vi "2. OCR.vi"() -> ()   [LabVIEW 2019]
doc: "c 2020 ReMiSYS All rights reserved."
panel:
  out "Image 2":T1(plugin-control)
  out "Data":string
  out "Image":T1(plugin-control)
  in  "Stop Button":bool
  # "c 2021 ReMiSYS All rights reserved."
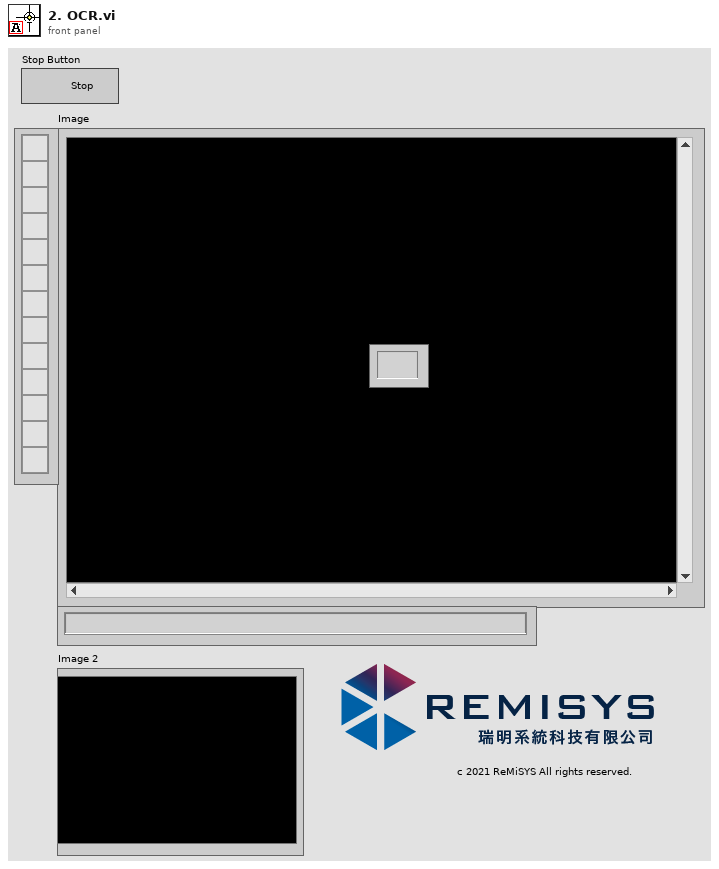
[diagram p1: front panel]
types:
  T1 = typedef "IMAQ Image.ctl" = refnum<image>
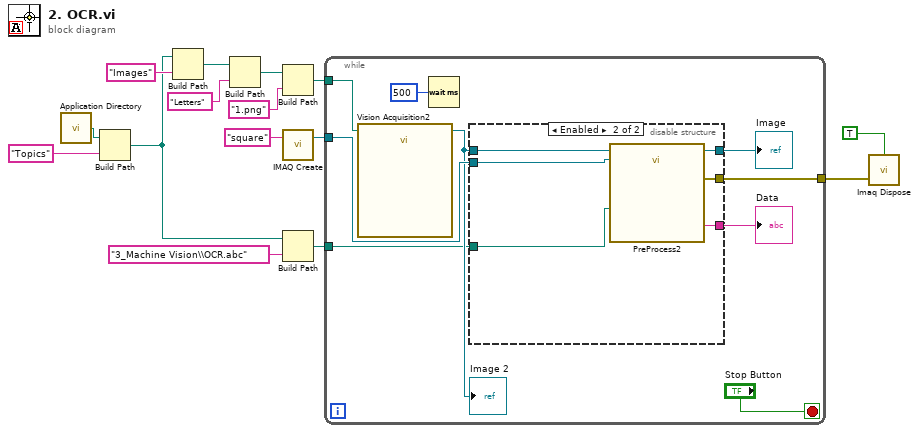
[diagram p0: block diagram]
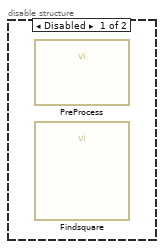
[diagram p2: hidden frame]
diagram:
  n1 = call <vilib>:"Application Directory.vi"() -> ("Application Directory"=w4:path)
  n2 = Build Path(base path=w4, name or relative path="Topics") -> (appended path=w1:path)
  n3 = Build Path(base path=w1, name or relative path="Images") -> (appended path=w8:path)
  n4 = Build Path(base path=w8, name or relative path="Letters") -> (appended path=w10:path)
  n5 = Build Path(base path=w10, name or relative path="1.png") -> (appended path=w9:path)
  n6 = call "IMAQ Create"("Image Name"="square") -> ("New Image"=w6:T1)  [unwired: 4 in, 1 out]
  n7 = Build Path(base path=w1, name or relative path="3_Machine Vision\\OCR.abc") -> (appended path=w2:path)
  n8 = while {
    tunnel: w9 -> [w24]
    tunnel: w6 -> [w21]
    tunnel: [w18] -> w5
    tunnel: w2 -> [w16]
    stop <- "Stop Button" stop-if-true
    n9 = call "Vision Acquisition2"("Image Path"=w24) -> ("Image Out"=w17:T1)  [unwired: 2 in, 24 out]
    "Image 2" <- w17
    n10 = Wait (ms)(milliseconds to wait=u32 500) -> ()  [unwired: 1 out]
    n11 = disable-structure shown="Enabled" {
      disable-tunnel: w17 -> [_ w30]
      disable-tunnel: w21 -> [_ w29]
      disable-tunnel: [_ w28] -> w20
      disable-tunnel: [_ w27] -> w19
      disable-tunnel: [_ w26] -> w18
      disable-tunnel: w16 -> [_ w25]
      frame Disabled {
        n12 = call "PreProcess"() -> ()  [unwired: 26 in, 2 out]
        n13 = call "Findsquare"() -> ()  [unwired: 24 in, 4 out]
      }
      frame Enabled {
        n14 = call "PreProcess2"("Image In"=w30, "Image Dst"=w29, "File Path (OCR/OCV 1)"=w25) -> ("Image Out"=w28:T1, "String (OCR/OCV 1)"=w27:string, "error out"=w26:errorcluster)  [unwired: 22 in]
      }
    }
    "Data" <- w19
    "Image" <- w20
  }
  n15 = call "Imaq Dispose"("All Images? (No)"=TRUE, "error in (no error)"=w5) -> ()  [unwired: 4 in, 1 out]
